vi "GC EX Vacuum - Step 2.vi"(7 "Step":i32, 8 "error in":errorcluster, 9 "Test Results In":T8, 10 "Gas":T1, 11 "GC Configuration":T2) -> (0 "error out":errorcluster, 1 "Test Results Out":T8, 2 "Gas Out":T1 caption="Gas", 3 "GC Configuration Out":T2)   [LabVIEW 2015]
uses:
  Controls/Test Information.ctl
  Controls/Vacuum Test.ctl
  Controls/Test Timing.ctl
  Controls/Vaccum Thresholds.ctl
  Controls/Helium Test.ctl
  Controls/Helium Thresholds.ctl
  CAN Communication/Gas/Typedefs/Session Handle.ctl
  CAN Communication/Gas/Gas.lvclass
  Controls/Test Results.ctl
  Controls/Step Result.ctl
  SubVIs/Timing/Timing.lvlib
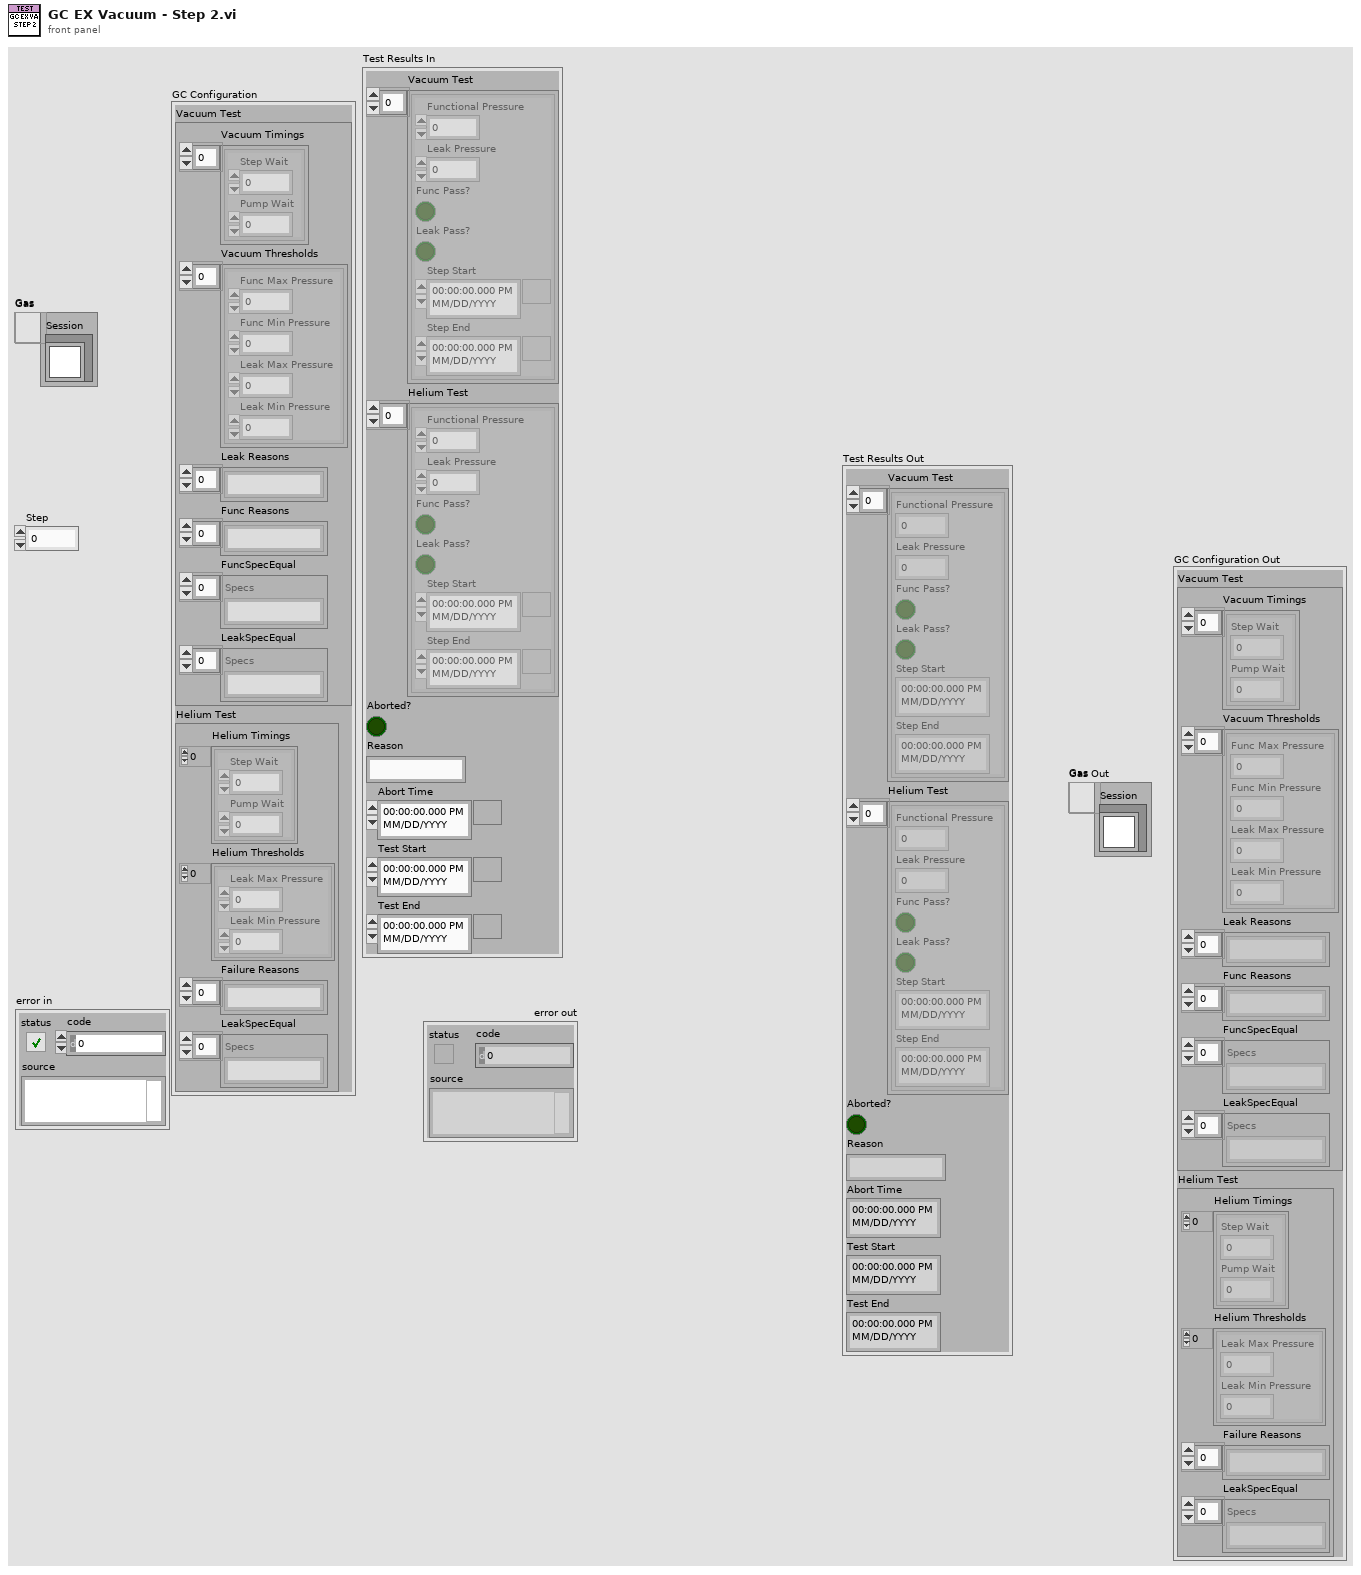
[diagram p1: front panel]
types:
  T1 = typedef "Gas.lvclass/Session Handle.ctl" = refnum<data-value>
  T2 = typedef "Test Information.ctl" = cluster{"Vacuum Test":T3, "Helium Test":T6}
  T3 = typedef "Vacuum Test.ctl" = cluster{"Vacuum Timings":T4[], "Vacuum Thresholds":T5[], "Leak Reasons":string[], "Func Reasons":string[], "FuncSpecEqual":string[], "LeakSpecEqual":string[]}
  T4 = typedef "Test Timing.ctl" = cluster{"Step Wait":dbl, "Pump Wait":dbl}
  T5 = typedef "Vaccum Thresholds.ctl" = cluster{"Func Max Pressure":dbl, "Func Min Pressure":dbl, "Leak Max Pressure":dbl, "Leak Min Pressure":dbl}
  T6 = typedef "Helium Test.ctl" = cluster{"Helium Timings":T4[], "Helium Thresholds":T7[], "Failure Reasons":string[], "LeakSpecEqual":string[]}
  T7 = typedef "Helium Thresholds.ctl" = cluster{"Leak Max Pressure":dbl, "Leak Min Pressure":dbl}
  T8 = typedef "Test Results.ctl" = cluster{"Vacuum Test":T9[], "Helium Test":T9[], "Aborted?":bool, "Reason":string, "Abort Time":timestamp, "Test Start":timestamp, "Test End":timestamp}
  T9 = typedef "Step Result.ctl" = cluster{"Functional Pressure":dbl, "Leak Pressure":dbl, "Func Pass?":bool, "Leak Pass?":bool, "Step Start":timestamp, "Step End":timestamp}
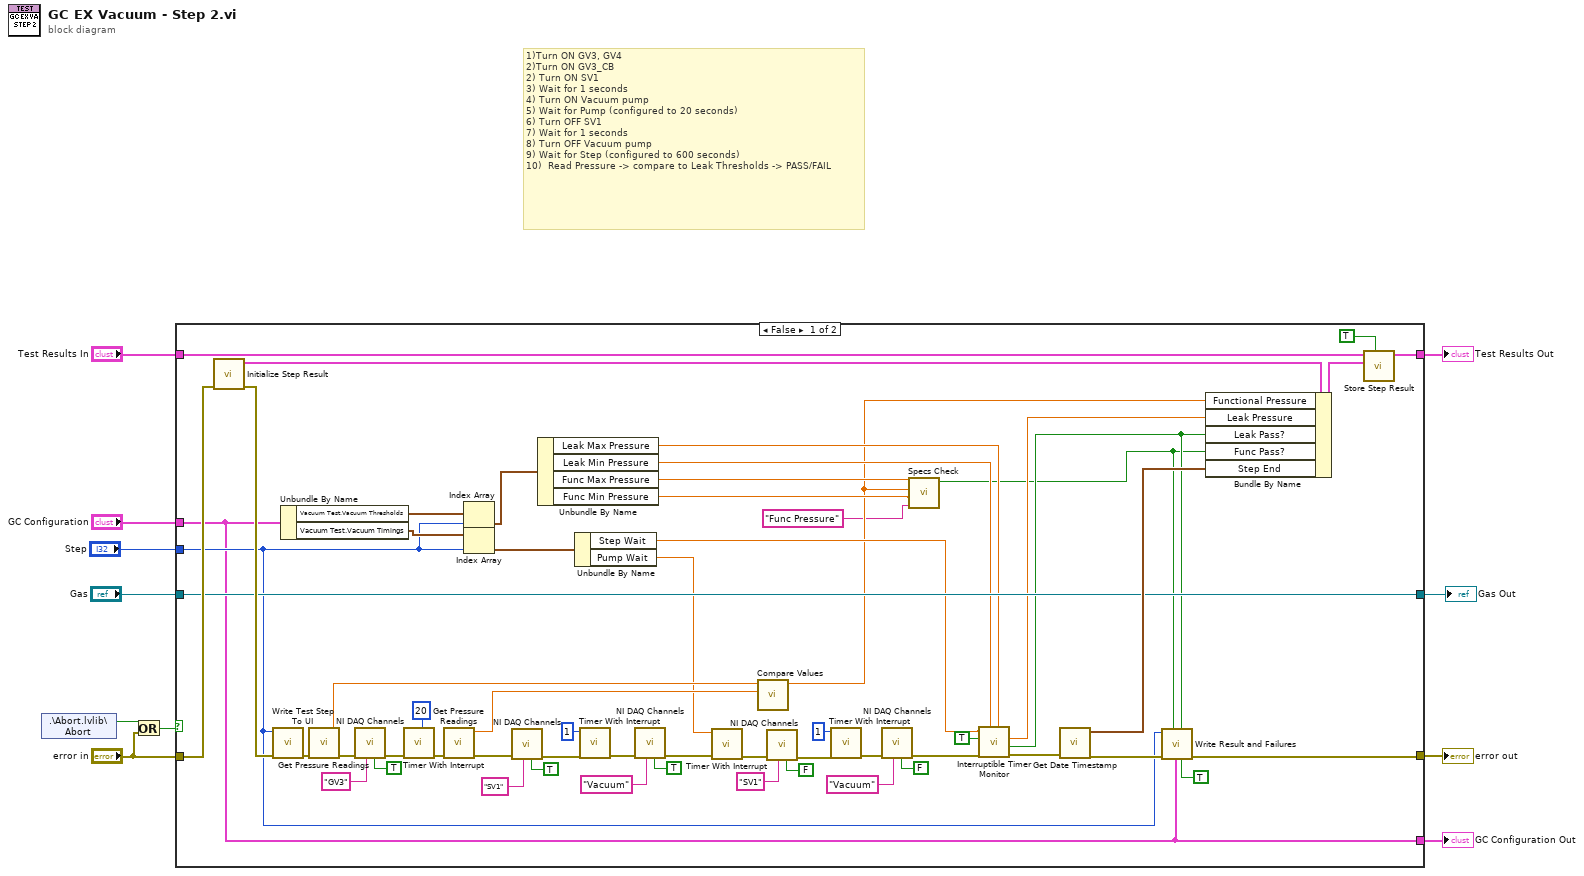
[diagram p0: block diagram]
diagram:
  # "1)Turn ON GV3, GV4\n2)Turn ON GV3_CB\n2) Turn ON SV1\n3) Wait for 1 seconds\n4) Turn ON Vacuum pump\n5) Wait for Pump (configured to 20 seconds)\n6) Turn OFF SV1\n7) Wait for 1 seconds\n8) Turn OFF Vacuum pump\n9) Wait for Step (configured to 600 seconds)\n10)  Read Pressure -> compare to Leak Thresholds -> PASS/FAIL"
  n1 = shared-variable ".\\Abort.lvlib\\Abort"() -> (w10:bool)  [unwired: 1 in, 1 out]
  n2 = Or(x=w10, y="error in") -> (x .or. y?=w9:bool)
  n3 = case shown="False" w9 {
    tunnel: "error in" -> [w69 w72]
    tunnel: "Test Results In" -> [w66 w73]
    tunnel: [w67 w73] -> w7
    tunnel: [w55 w72] -> w6
    tunnel: "GC Configuration" -> [w53 w71]
    tunnel: "Step" -> [w54 _]
    tunnel: [w53 w71] -> w3
    tunnel: [w59 w70] -> w1
    tunnel: "Gas" -> [w59 w70]
    frame False {
      n4 = call "Initialize Step Result.vi"("error in (no error)"=w69) -> ("error out"=w68:errorcluster, "New Step Result"=w65:T9)  [unwired: 8 in, 1 out]
      n5 = call "Write Test Step To UI.vi"("error in (no error)"=w68, "Step"=w54) -> ("error out"=w46:errorcluster)  [unwired: 9 in]
      n6 = Unbundle By Name(w53) -> ("Vacuum Test.Vacuum Thresholds"=w62:T5[], "Vacuum Test.Vacuum Timings"=w61:T4[])
      n7 = call "Get Pressure Readings.vi"("error in (no error)"=w46) -> ("error out"=w43:errorcluster, "NI-DAQ Pressure"=w51:dbl)  [unwired: 6 in, 3 out]
      n8 = call "NI DAQ Channels.vi"("Control"=TRUE ("State"), "Channel"="GV3", "error in (no error)"=w43) -> ("error out"=w42:errorcluster)  [unwired: 7 in, 1 out]
      n9 = call "Timer With Interrupt.vi"("error in (no error)"=w42, "Wait (s)"=20) -> ("error out"=w50:errorcluster)  [unwired: 7 in, 2 out]
      n10 = call "Get Pressure Readings.vi"("error in (no error)"=w50) -> ("error out"=w40:errorcluster, "NI-DAQ Pressure"=w52:dbl)  [unwired: 6 in, 3 out]
      n11 = Index Array(array=w62, index=w54) -> (element=w57:T5)
      n12 = Index Array(array=w61, index=w54) -> (element=w60:T4)
      n13 = call "NI DAQ Channels.vi"("Control"=TRUE ("State"), "Channel"="SV1", "error in (no error)"=w40) -> ("error out"=w39:errorcluster)  [unwired: 7 in, 1 out]
      n14 = Unbundle By Name(w57) -> ("Leak Max Pressure"=w24:dbl, "Leak Min Pressure"=w25:dbl, "Func Max Pressure"=w16:dbl, "Func Min Pressure"=w15:dbl)
      n15 = Unbundle By Name(w60) -> ("Step Wait"=w27:dbl, "Pump Wait"=w48:dbl)
      n16 = call "Timer With Interrupt.vi"("error in (no error)"=w39, "Wait (s)"=1) -> ("error out"=w37:errorcluster)  [unwired: 7 in, 2 out]
      n17 = call "NI DAQ Channels.vi"("Control"=TRUE ("State"), "Channel"="Vacuum", "error in (no error)"=w37) -> ("error out"=w36:errorcluster)  [unwired: 7 in, 1 out]
      n18 = call "Timer With Interrupt.vi"("error in (no error)"=w36, "Wait (s)"=w48) -> ("error out"=w34:errorcluster)  [unwired: 7 in, 2 out]
      n19 = call "Compare Values.vi"("P2"=w52, "P1"=w51) -> ("Abs Diff"=w14:dbl)  [unwired: 9 in]
      n20 = call "NI DAQ Channels.vi"("Control"=FALSE ("State"), "Channel"="SV1", "error in (no error)"=w34) -> ("error out"=w33:errorcluster)  [unwired: 7 in, 1 out]
      n21 = call "Timer With Interrupt.vi"("error in (no error)"=w33, "Wait (s)"=1) -> ("error out"=w31:errorcluster)  [unwired: 7 in, 2 out]
      n22 = call "NI DAQ Channels.vi"("Control"=FALSE ("State"), "Channel"="Vacuum", "error in (no error)"=w31) -> ("error out"=w29:errorcluster)  [unwired: 7 in, 1 out]
      n23 = call "Specs Check.vi"("parameter"="Func Pressure", "lower limit"=w15, "x"=w14, "upper limit"=w16) -> ("In Range?"=w13:bool)  [unwired: 6 in, 1 out]
      n24 = call "Interruptible Timer Monitor.vi"("Max"=w24, "Min"=w25, "error in (no error)"=w29, "Update UI?"=TRUE, "Wait (s)"=w27) -> ("error out"=w28:errorcluster, "In Range?"=w22:bool, "Leak Rate"=w23:dbl)  [unwired: 2 in, 2 out]
      n25 = call "Get Date Timestamp.vi"("error in (no error)"=w28) -> ("error out"=w56:errorcluster, "current time"=w63:timestamp)  [unwired: 9 in]
      n26 = call "Write Result and Failures.vi"("Vacuum?"=TRUE, "Leak"=w22, "GC Configuration"=w53, "Func"=w13, "error in (no error)"=w56, "Step"=w54) -> ("error out"=w55:errorcluster)  [unwired: 5 in]
      n27 = Bundle By Name(cluster=w65, "Functional Pressure"=w14, "Leak Pressure"=w23, "Leak Pass?"=w22, "Func Pass?"=w13, "Step End"=w63) -> (w64:T9)
      n28 = call "Store Step Result.vi"("Vacuum?"=TRUE, "Step Result"=w64, "Test Results In"=w66) -> ("Test Results Out"=w67:T8)  [unwired: 8 in]
    }
    frame True {
    }
  }
  "error out" <- w6
  "Test Results Out" <- w7
  "GC Configuration Out" <- w3
  "Gas Out" <- w1
